vi "DataReadTxtFileMod.vi"(6 "VarParIndex":i32, 8 "error in":errorcluster, 9 "ScanlistIndex":i32, 10 "chemin Data":path, 11 "Chemin Header":path) -> (0 "error out":errorcluster, 1 "Y Array":dbl[](array[numeric]), 2 "X Array":dbl[](array[numeric]), 3 "Data Preview":string[][](array[string]), 4 "CurveName":string, 5 "VarPar":string, 7 "Header String":string)   [LabVIEW 2019]
doc: "Ce VI lit les données contenu dans le fichier de sauvegarde automatique. Ces données correspondent aux valeurs prises lors du dernier balayage. La sauvegarde automatique est effectué après chaque acquisition."
uses:
  Interface Class/ScanParams.ctl
  Interface Class/ScanParamsOld.ctl
  Interface Class/Interface.lvclass
panel:
  out "x = y ?":bool
  out "enregistrement(s)":T1={"Entête"="", "Scan list"=[], "NbCourbe"=1, "IndCourbe"=0, "NomDon"=["RTêta;", "X&Y;"], "Session "=0, "Date"="", "Time"="", "VarParams"=[], "UserName"="", "ScanTableSize"=[], "VarPar list"=[], "DescKeyword"=""} caption="ScanParams"
  out "AllData":dbl[][](array[numeric]) format="%#.16f"
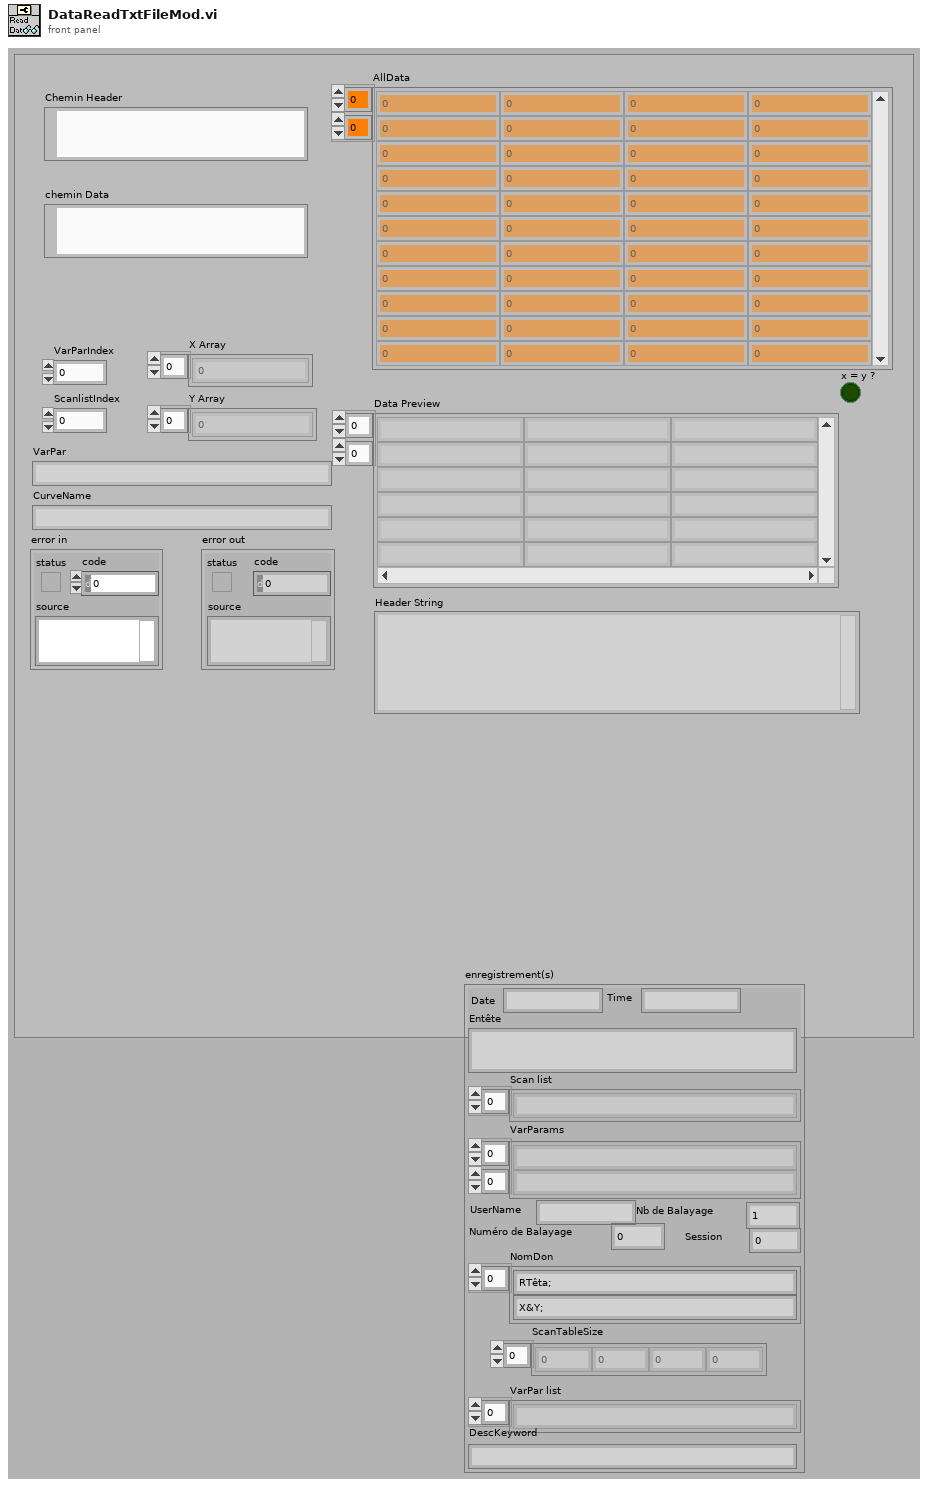
[diagram p1: front panel]
types:
  T1 = typedef "Interface.lvclass/ScanParams.ctl" = cluster{"Entête":string, "Scan list":string[], "NbCourbe":i32, "IndCourbe":i64, "NomDon":string[], "Session ":i32, "Date":string, "Time":string, "VarParams":string[][], "UserName":string, "ScanTableSize":i32[], "VarPar list":string[], "DescKeyword":string}
  T2 = typedef "Interface.lvclass/ScanParamsOld.ctl" = cluster{"Entête":string, "Scan list":string[], "NbCourbe":i32, "IndCourbe":i64, "NomDon":string[], "Session ":i32, "Date":string, "Time":string, "VarParams":string[][], "UserName":string, "ScanTableSize":i32[], "VarPar list":string[]}
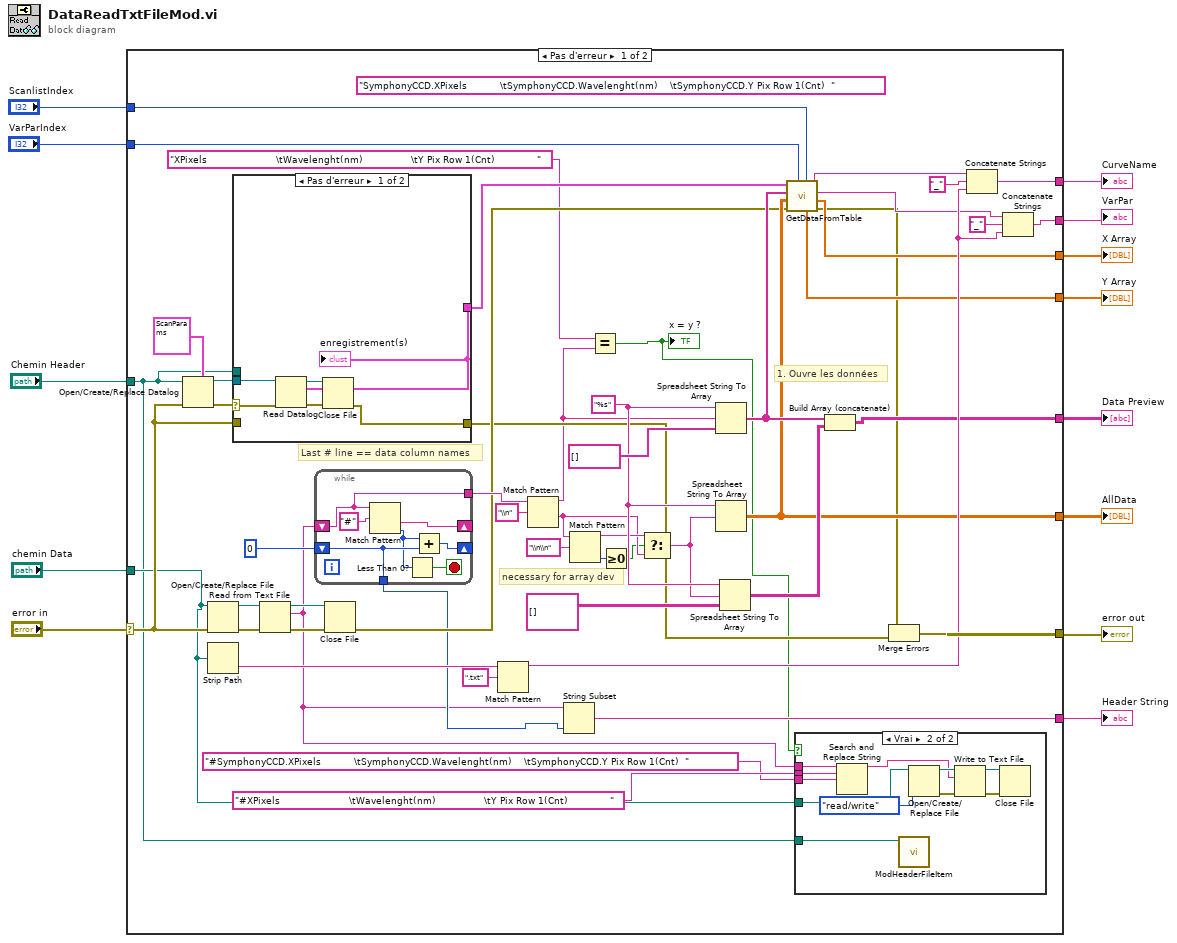
[diagram p0: block diagram]
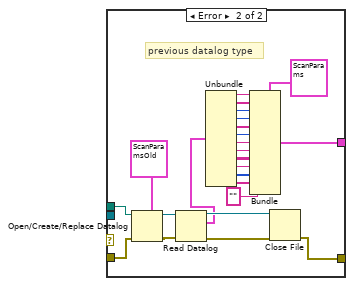
[diagram p3: hidden frame]
diagram:
  n1 = case shown="Pas d'erreur" "error in" {
    selector: "error in" -> [w32 w114]
    tunnel: "chemin Data" -> [w16 _]
    tunnel: [w34 w114] -> w13
    tunnel: [w48 _] -> w10
    tunnel: [w45 _] -> w9
    tunnel: "Chemin Header" -> [w14 _]
    tunnel: "ScanlistIndex" -> [w36 _]
    tunnel: "VarParIndex" -> [w38 _]
    tunnel: [w42 _] -> w5
    tunnel: [w41 _] -> w4
    tunnel: [w53 _] -> w3
    tunnel: [w55 _] -> w2
    tunnel: [w30 _] -> w1
    frame No Error {
      (unwired) "SymphonyCCD.XPixels           \tSymphonyCCD.Wavelenght(nm)    \tSymphonyCCD.Y Pix Row 1(Cnt)  " ("chaîne de format")
      w50 = "%s" ("chaîne de format")
      # "necessary for array dev"
      # "Last # line == data column names"
      # "1. Ouvre les données"
      n2 = Open/Create/Replace Datalog(5:T1 {"Entête"="", "Scan list"=[], "NbCourbe"=1, "IndCourbe"=1, "NomDon"=["RTêta;", "X&Y;"], "Session "=0, "Date"="", "Time"="", "VarParams"=[], "UserName"="", "ScanTableSize"=[], "VarPar list"=[], "DescKeyword"=""} ("ScanParams"), 8:w32, 11:w14) -> (0:w35:errorcluster, 3:w58:refnum<k1>)  [unwired: 3 in, 1 out]
      n3 = Open/Create/Replace File(file path (use dialog)=w16, error in=w32) -> (refnum out=w65:refnum<file>, error out=w64:errorcluster)  [unwired: 4 in, 1 out]
      n4 = Strip Path(path=w16) -> (name=w57:string)  [unwired: 1 out]
      n5 = case shown="Pas d'erreur" w35 {
        selector: w35 -> [w78 _]
        tunnel: w58 -> [w82 _]
        tunnel: [w79 w84] -> w37
        tunnel: w14 -> [_ w101]
        tunnel: [w77 w85] -> w33
        tunnel: w32 -> [_ w83]
        frame No Error {
          n6 = Read Datalog(4:w78, 7:w82) -> (0:w81:errorcluster, 2:w79:T1, 3:w80:refnum<k1>)  [unwired: 1 in]
          "enregistrement(s)" <- w79
          n7 = Close File(refnum=w80, error in=w81) -> (error out=w77:errorcluster)  [unwired: 1 out]
        }
        frame Error {
          # "previous datalog type"
          n8 = Open/Create/Replace Datalog(5:T2 {"Entête"="", "Scan list"=[], "NbCourbe"=1, "IndCourbe"=1, "NomDon"=["RTêta;", "X&Y;"], "Session "=0, "Date"="", "Time"="", "VarParams"=[], "UserName"="", "ScanTableSize"=[], "VarPar list"=[]} ("ScanParams"), 8:w83, 11:w101) -> (0:w103:errorcluster, 3:w104:refnum<k1>)  [unwired: 3 in, 1 out]
          n9 = Read Datalog(4:w103, 7:w104) -> (0:w106:errorcluster, 2:w100:T2, 3:w105:refnum<k1>)  [unwired: 1 in]
          n10 = Unbundle(w100) -> ("Entête"=w98:string, "Scan list"=w97:string[], "NbCourbe"=w96:i32, "IndCourbe"=w95:i64, "NomDon"=w94:string[], "Session"=w93:i32, "Date"=w92:string, "Time"=w91:string, "VarParams"=w90:string[][], "UserName"=w89:string, "ScanTableSize"=w88:i32[], "VarPar list"=w87:string[])
          n11 = Bundle(cluster=T1 {"Entête"="", "Scan list"=[], "NbCourbe"=1, "IndCourbe"=1, "NomDon"=["RTêta;", "X&Y;"], "Session "=0, "Date"="", "Time"="", "VarParams"=[], "UserName"="", "ScanTableSize"=[], "VarPar list"=[], "DescKeyword"=""} ("ScanParams"), "Entête"=w98, "Scan list"=w97, "NbCourbe"=w96, "IndCourbe"=w95, "NomDon"=w94, "Session"=w93, "Date"=w92, "Time"=w91, "VarParams"=w90, "UserName"=w89, "ScanTableSize"=w88, "VarPar list"=w87, "DescKeyword"="") -> (w84:T1)
          n12 = Close File(refnum=w105, error in=w106) -> (error out=w85:errorcluster)  [unwired: 1 out]
        }
      }
      n13 = Read from Text File(file (use dialog)=w65, error in=w64) -> (refnum out=w62:refnum<file>, text=w17:string, error out=w63:errorcluster)  [unwired: 2 in, 1 out]
      n14 = while {
        shift-right: [w112] -> _
        shift-left: w17 -> [w110]
        tunnel: [w110] -> w61
        shift-right: [w107] -> _
        shift-left: 0 ("offset past match") -> [w109]
        tunnel: [w109] -> w28
        stop <- w111 stop-if-true
        n15 = Match Pattern(string=w110, regular expression="#" ("expression régulière")) -> (after substring=w112:string, offset past match=w108:i32)  [unwired: 1 in, 2 out]
        n16 = Less Than 0?(x=w108) -> (x < 0?=w111:bool)
        n17 = Add(x=w108, y=w109) -> (x+y=w107:i32)
      }
      n18 = Close File(refnum=w62, error in=w63) -> (error out=w39:errorcluster)  [unwired: 1 out]
      n19 = Match Pattern(string=w57, regular expression=".txt" ("expression régulière")) -> (before substring=w52:string)  [unwired: 1 in, 3 out]
      n20 = Match Pattern(string=w61, regular expression="\\n" ("expression régulière")) -> (before substring=w21:string, after substring=w24:string)  [unwired: 1 in, 2 out]
      n21 = String Subset(string=w17, length (rest)=w28) -> (substring=w30:string)  [unwired: 1 in]
      n22 = Match Pattern(string=w24, regular expression="\\n\\n" ("expression régulière")) -> (before substring=w26:string, offset past match=w22:i32)  [unwired: 1 in, 2 out]
      n23 = Equal?(x="XPixels                       \tWavelenght(nm)                \tY Pix Row 1(Cnt)              " ("chaîne de format"), y=w21) -> (x = y?=w15:bool)
      "x = y ?" <- w15
      n24 = Greater Or Equal To 0?(x=w22) -> (x >= 0?=w23:bool)
      n25 = Select(t=w26, s=w23, f=w24) -> (s? t:f=w25:string)
      n26 = Spreadsheet String To Array(format string=w50, spreadsheet string=w21, array type (2D Dbl)=string[] []) -> (array=w46:string[])  [unwired: 1 in]
      n27 = Spreadsheet String To Array(format string=w50, spreadsheet string=w25) -> (array=w45:dbl[][])  [unwired: 2 in]
      n28 = Spreadsheet String To Array(format string=w50, spreadsheet string=w25, array type (2D Dbl)=string[][] []) -> (array=w49:string[][])  [unwired: 1 in]
      n29 = call "GetDataFromTable.vi"("ScanlistIndex"=w36, "VarParIndex"=w38, "error in"=w39, "AllDataIn"=w45, "FilesColName"=w46, "DataRecord"=w37) -> ("error out"=w40:errorcluster, "X Array"=w41:dbl[], "VarPar"=w43:string, "CurveName"=w44:string, "Y Array"=w42:dbl[])  [unwired: 1 in]
      n30 = case shown="Vrai" w15 {
        tunnel: "#XPixels                       \tWavelenght(nm)                \tY Pix Row 1(Cnt)              " ("chaîne de format") -> [_ w76]
        tunnel: "#SymphonyCCD.XPixels           \tSymphonyCCD.Wavelenght(nm)    \tSymphonyCCD.Y Pix Row 1(Cnt)  " ("chaîne de format") -> [_ w75]
        tunnel: w17 -> [_ w74]
        tunnel: w16 -> [_ w73]
        tunnel: w14 -> [_ w66]
        frame False {
        }
        frame True {
          n31 = Search and Replace String(input string=w74, search string=w76, replace string=w75) -> (result string=w71:string)  [unwired: 5 in, 3 out]
          n32 = call "ModHeaderFileItem.vi"("Data Path"=w66) -> ()  [unwired: 10 in, 1 out]
          n33 = Open/Create/Replace File(file path (use dialog)=w73, access (0:read/write)=enum16{"read/write", "read-only", "write-only"}."read/write" ("accès (0 : read/write)")) -> (refnum out=w72:refnum<file>, error out=w70:errorcluster)  [unwired: 4 in, 1 out]
          n34 = Write to Text File(file (use dialog)=w72, text=w71, error in=w70) -> (refnum out=w68:refnum<file>, error out=w67:errorcluster)  [unwired: 1 in, 1 out]
          n35 = Close File(refnum=w68, error in=w67) -> ()  [unwired: 2 out]
        }
      }
      n36 = Build Array (concatenate)(w46, w49) -> (w48:string[][])
      n37 = Merge Errors(w40, w33) -> (w34:errorcluster)
      n38 = Concatenate Strings(w44, "_" ("chaîne"), w52) -> (w55:string)
      n39 = Concatenate Strings(w43, "_" ("chaîne"), w52) -> (w53:string)
    }
    frame Error {
    }
  }
  "error out" <- w13
  "Data Preview" <- w10
  "AllData" <- w9
  "Y Array" <- w5
  "X Array" <- w4
  "VarPar" <- w3
  "CurveName" <- w2
  "Header String" <- w1
